vi "Wiimote Close.vi"(8 "error in (no error)":errorcluster, 11 "LV WiiMote Interface":T1) -> (0 "error out":errorcluster)   [LabVIEW 2012, in "LV Wiimote Interface.lvclass"]
uses:
  LV Wiimote Interface.lvclass
  Controls/LV Wiimote Interface.ctl
  LV Wiimote Interface.lvclass/LV Wiimote Interface.ctl
  C:/Program Files/National Instruments/LabVIEW 2012/vi.lib/LabVIEW Hacker/WiiMote/Dependencies/WiimoteLib.dll
  Program Files/National Instruments/LabVIEW 2012/vi.lib/LabVIEW Hacker/WiiMote/Dependencies/WiimoteLib.dll
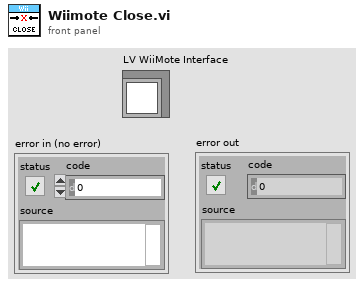
[diagram p1: front panel]
types:
  T1 = typedef "LV Wiimote Interface.ctl" = refnum<class "LV Wiimote Interface.lvclass">
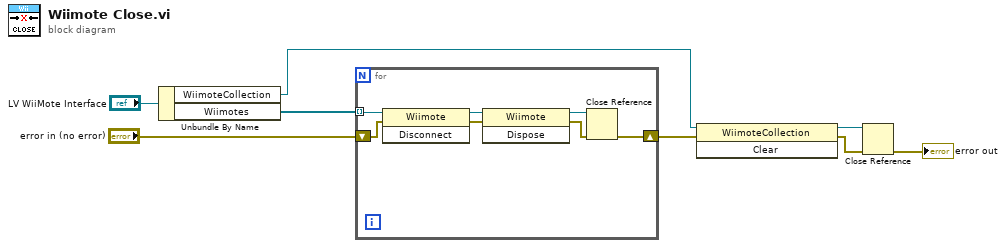
[diagram p0: block diagram]
diagram:
  n1 = Unbundle By Name("LV WiiMote Interface") -> ("WiimoteCollection"=w4:refnum<k24>, "Wiimotes"=w7:refnum<k24>[])
  n2 = for {
    tunnel: w7 -> [w15] mode=indexing
    shift-right: [w9] -> w5
    shift-left: "error in (no error)" -> [w10]
    n3 = invoke class="Wiimote" method="Disconnect"(reference=w15, error in=w10) -> (reference out=w14:refnum<k24>, error out=w13:errorcluster)  [unwired: 1 in, 1 out]
    n4 = invoke class="Wiimote" method="Dispose"(reference=w14, error in=w13) -> (reference out=w12:refnum<k24>, error out=w11:errorcluster)  [unwired: 1 in, 1 out]
    n5 = Close Reference(reference=w12, error in (no error)=w11) -> (error out=w9:errorcluster)
  }
  n6 = invoke class="WiimoteCollection" method="Clear"(reference=w4, error in=w5) -> (reference out=w3:refnum<k24>, error out=w2:errorcluster)  [unwired: 1 in, 1 out]
  n7 = Close Reference(reference=w3, error in (no error)=w2) -> (error out=→"error out":errorcluster)
